vi "Convert Dataset to Strings.vi"(9 "Projectile Velocity (Meters/Second)":dbl format="%_4g", 10 "X Values (Seconds)":dbl[](array[numeric]), 11 "Y Values (Voltage)":dbl[](array[numeric])) -> (2 "DataSet Rows":string[](array[string]))   [LabVIEW 2021]
doc: "Converts dataset into strings, and prepends a column header."
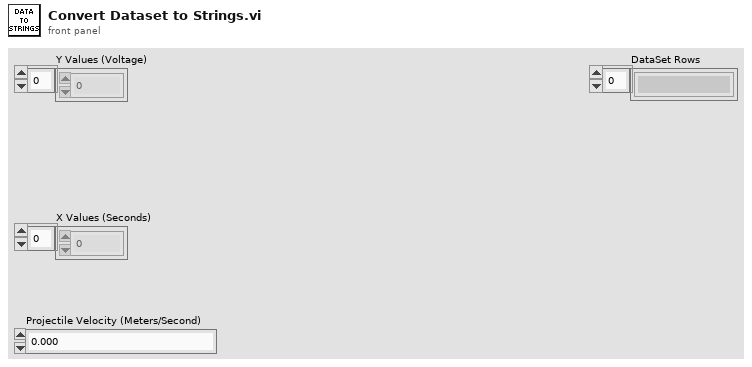
[diagram p1: front panel]
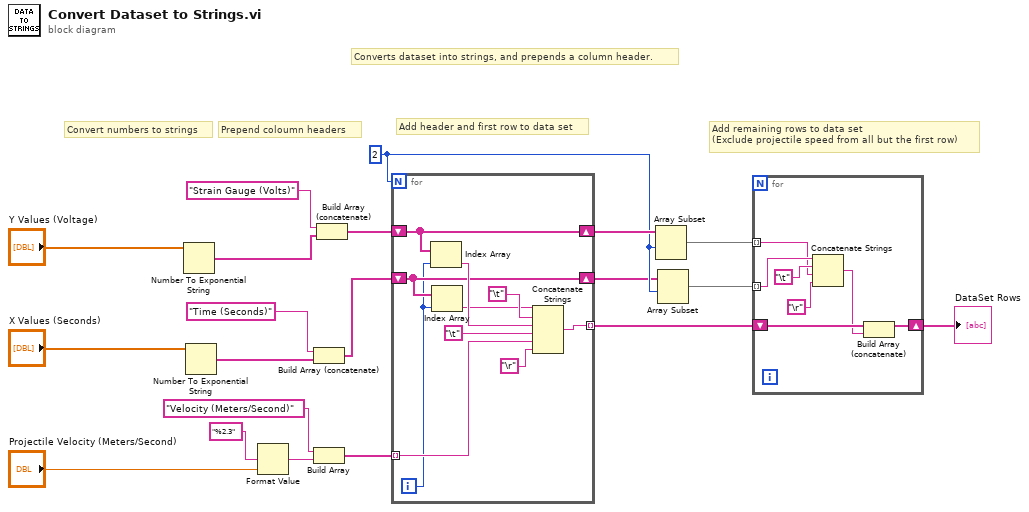
[diagram p0: block diagram]
diagram:
  w5 = 2
  # "Add remaining rows to data set\n(Exclude projectile speed from all but the first row)"
  # "Add header and first row to data set"
  # "Convert numbers to strings"
  # "Prepend coloumn headers"
  # "Converts dataset into strings, and prepends a column header."
  n1 = Number To Exponential String(number="Y Values (Voltage)") -> (E-format string=w18:string[])  [unwired: 3 in]
  n2 = Number To Exponential String(number="X Values (Seconds)") -> (E-format string=w15:string[])  [unwired: 3 in]
  n3 = Format Value(format string="%2.3", value (0)="Projectile Velocity (Meters/Second)") -> (output string=w12:string)  [unwired: 1 in]
  n4 = Build Array (concatenate)("Time (Seconds)", w15) -> (w9:string[])
  n5 = Build Array("Velocity (Meters/Second)" ("element"), w12) -> (w10:string[])
  n6 = Build Array (concatenate)("Strain Gauge (Volts)", w18) -> (w8:string[])
  n7 = for {
    N: w5 -> [_]
    tunnel: w10 -> [w28] mode=indexing
    tunnel: [w27] -> w7 mode=indexing
    shift-right: [w26] -> w6
    shift-left: w8 -> [w26]
    shift-right: [w24] -> w4
    shift-left: w9 -> [w24]
    i -> [w22]
    n8 = Index Array(array=w26, index=w22) -> (element=w25:string)
    n9 = Index Array(array=w24, index=w22) -> (element=w23:string)
    n10 = Concatenate Strings(w23, "\t", w25, "\t", w28, "\r") -> (w27:string)
  }
  n11 = Array Subset(array=w6, index=w5) -> (w2:string[])  [unwired: 1 in]
  n12 = Array Subset(array=w4, index=w5) -> (w3:string[])  [unwired: 1 in]
  n13 = for {
    tunnel: w3 -> [w36] mode=indexing
    tunnel: w2 -> [w34] mode=indexing
    shift-right: [w32] -> w1
    shift-left: w7 -> [w37]
    n14 = Concatenate Strings(w36, "\t", w34, "\r") -> (w33:string)
    n15 = Build Array (concatenate)(w37, w33) -> (w32:string[])
  }
  "DataSet Rows" <- w1
